vi "Bertta_v06_3.vi"() -> ()   [LabVIEW 2015]
uses:
  x64/Debug/BERTTA.dll
panel:
  in  "Tab Control":T1(tab)
  in  "Description":string
  in  "Project name":string
  in  "User (initials)":string
  out "PUMP 1":bool
  out "Mettler 5":dynamicdata(graph)
  out "Temp":dynamicdata(graph)
  out "Target":dbl
  out "Scale weight":dbl
  out "Amount now":dbl
  out "Flow rate":dbl
  out "Time to target":dbl format="%<%H:%M:%S>t"
  out "Current step":dbl
  out "weightcontrol":i32
  out "timecontrol":i32
  out "target_control":i32
  in  "Balances":bool[](array[boolean])
  out "Waveform Chart 3":dynamicdata(graph)
  out "Table":string[][](table)
  in  "Headers":string[](array[string])
  out "Boolean 12":bool
  out "Boolean 7":bool
  out "Boolean 6":bool
  out "Boolean 5":bool
  out "Boolean 4":bool
  in  "?":bool
  in  "Seq":dbl[][](array[numeric])=[[20.0, 45.0, 50.0], [46.0, 50.0, 20.0], [3.0, 3.0, 3.0]]
  out "T control":dbl
  out "Tr":dbl
  out "Tj in":dbl
  out "Tj out":dbl
  out "DT":dbl
  out "Current step":i32
  out "Elapsed":i32
  in  "Tbypass":dbl=20.0
  in  "Tfail":dbl=22.0
  in  "err":i32
  in  "PAUSE":bool
  out "Tinit":dbl
  out "Tset":dbl
  out "Time limit":dbl
  out "Waveform Chart":dynamicdata(graph)
  in  "Lauda port":dbl=9.0
  in  "Port":i32=10
  in  "Radio Buttons":enum32{"Reglo Digital", "Reglo Analog", "PAM"}(radio)
  out "Speed":dbl
  out "mA":dbl format="%#_2g"
  in  "Port":i32=15
  out "RPM":dbl format="%#_2g"
  out "Boolean 18":bool
  out "Boolean 17":bool
  out "Boolean 16":bool
  out "Boolean 15":bool
  out "Boolean 14":bool
  out "Boolean 13":bool
  out "Boolean 11":bool
  out "Boolean 10":bool
  out "Boolean 9":bool
  out "Boolean 8":bool
  in  "Seq 2":dbl[][](array[numeric])=[[3.0, 3.0, 7.0], [2.0, 2.0, 2.0], [4.0, 2.0, 100.0]]
  in  "?":bool
  out "Flow rate (g/min)":dbl
  out "Time (min)":dbl
  out "Target (g)":dbl
  out "Scale reading (g)":dbl
  out "Amount now (g)":dbl
  out "Time to target (min)":dbl format="%<%H:%M:%S>t"
  in  "Bypass (g/min)":dbl
  out "Waveform Chart 2":dynamicdata(graph)
  in  "?":bool
  out "RPM":dbl
  out "Torque":dbl
  in  "Set RPM":dbl(slide) scale=0.0..500.0
  out "Waveform Chart 4":dynamicdata(graph)
  in  "?":T2(tab)
  in  "Device port":dbl=13.0
  # "1"
  # "2"
  # "3"
  # "4"
  # "Tinit     >    Tset       min. time"
  # "Grams    /   min"
  # "Pump configuration"
  # "Scale configuration"
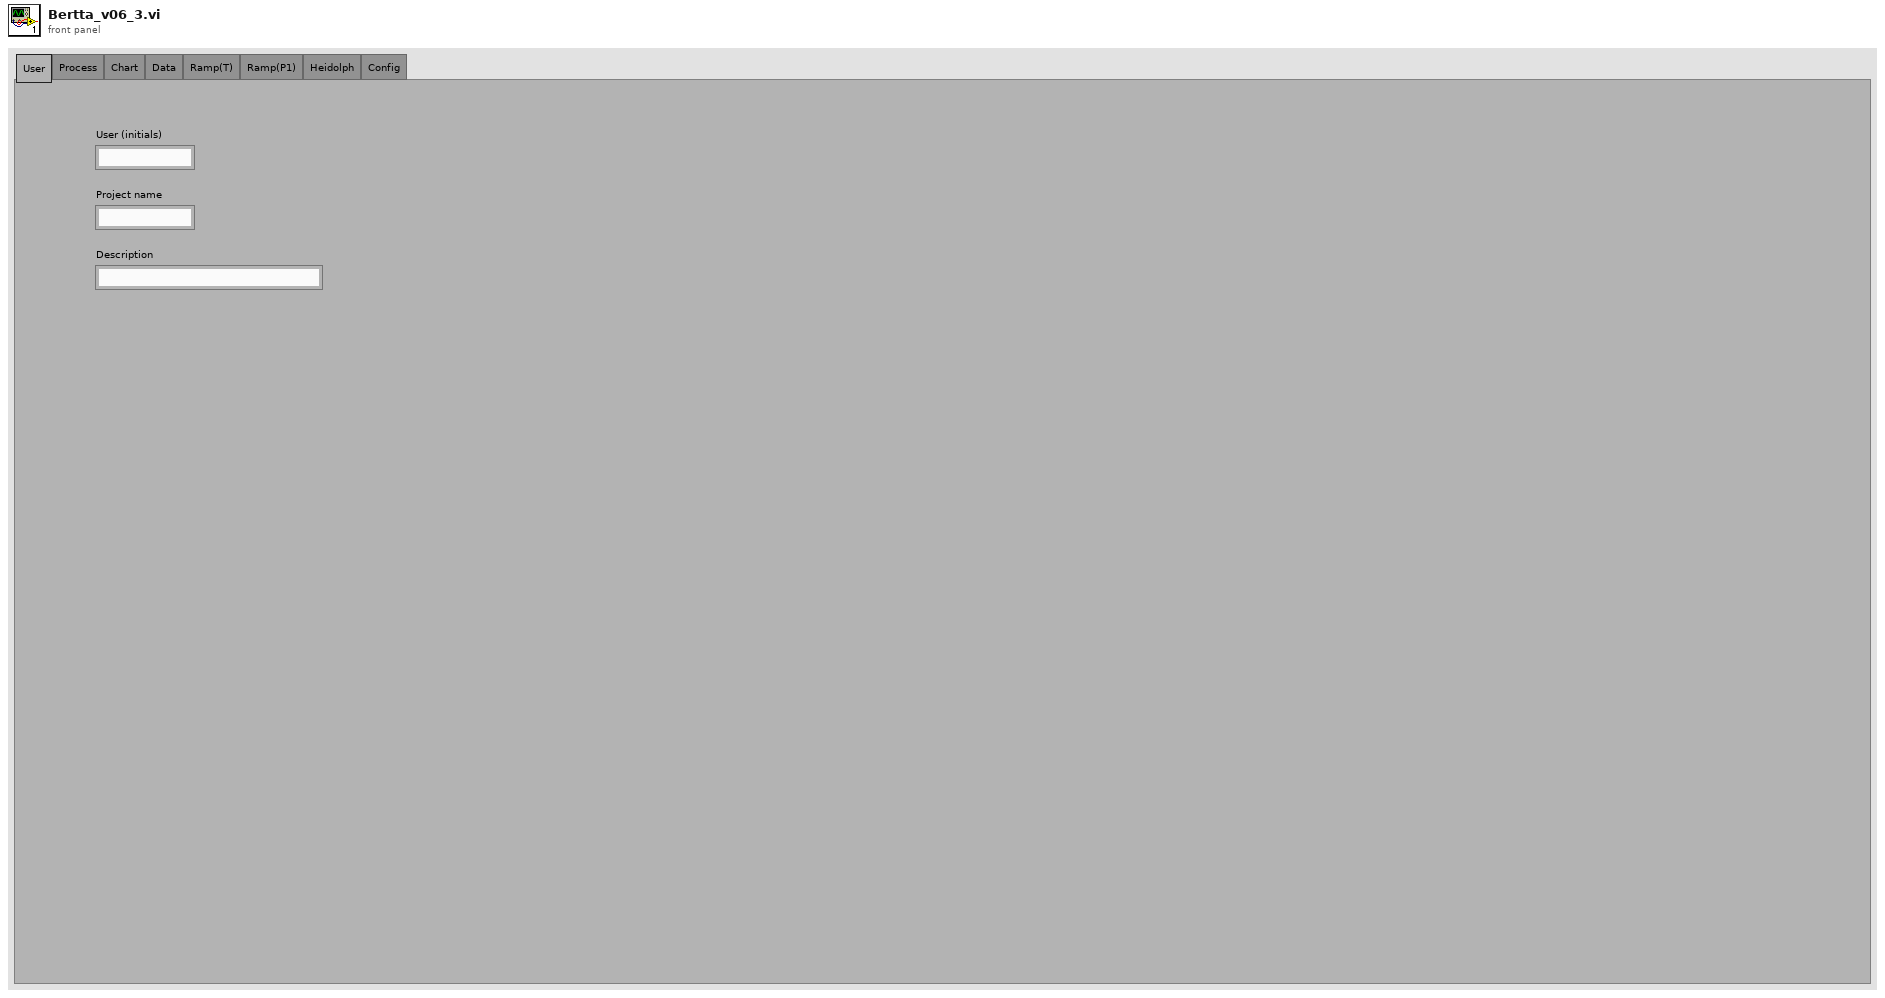
[diagram p1: front panel]
types:
  T1 = enum32{"User", "Process", "Chart", "Data", "Ramp(T)", "Ramp(P1)", "Heidolph", "Config"}
  T2 = enum32{"DB / File", "Lauda", "Heidolph", "Mettler 1", "Mettler 2", "Mettler 3", "Ismatec 1"}
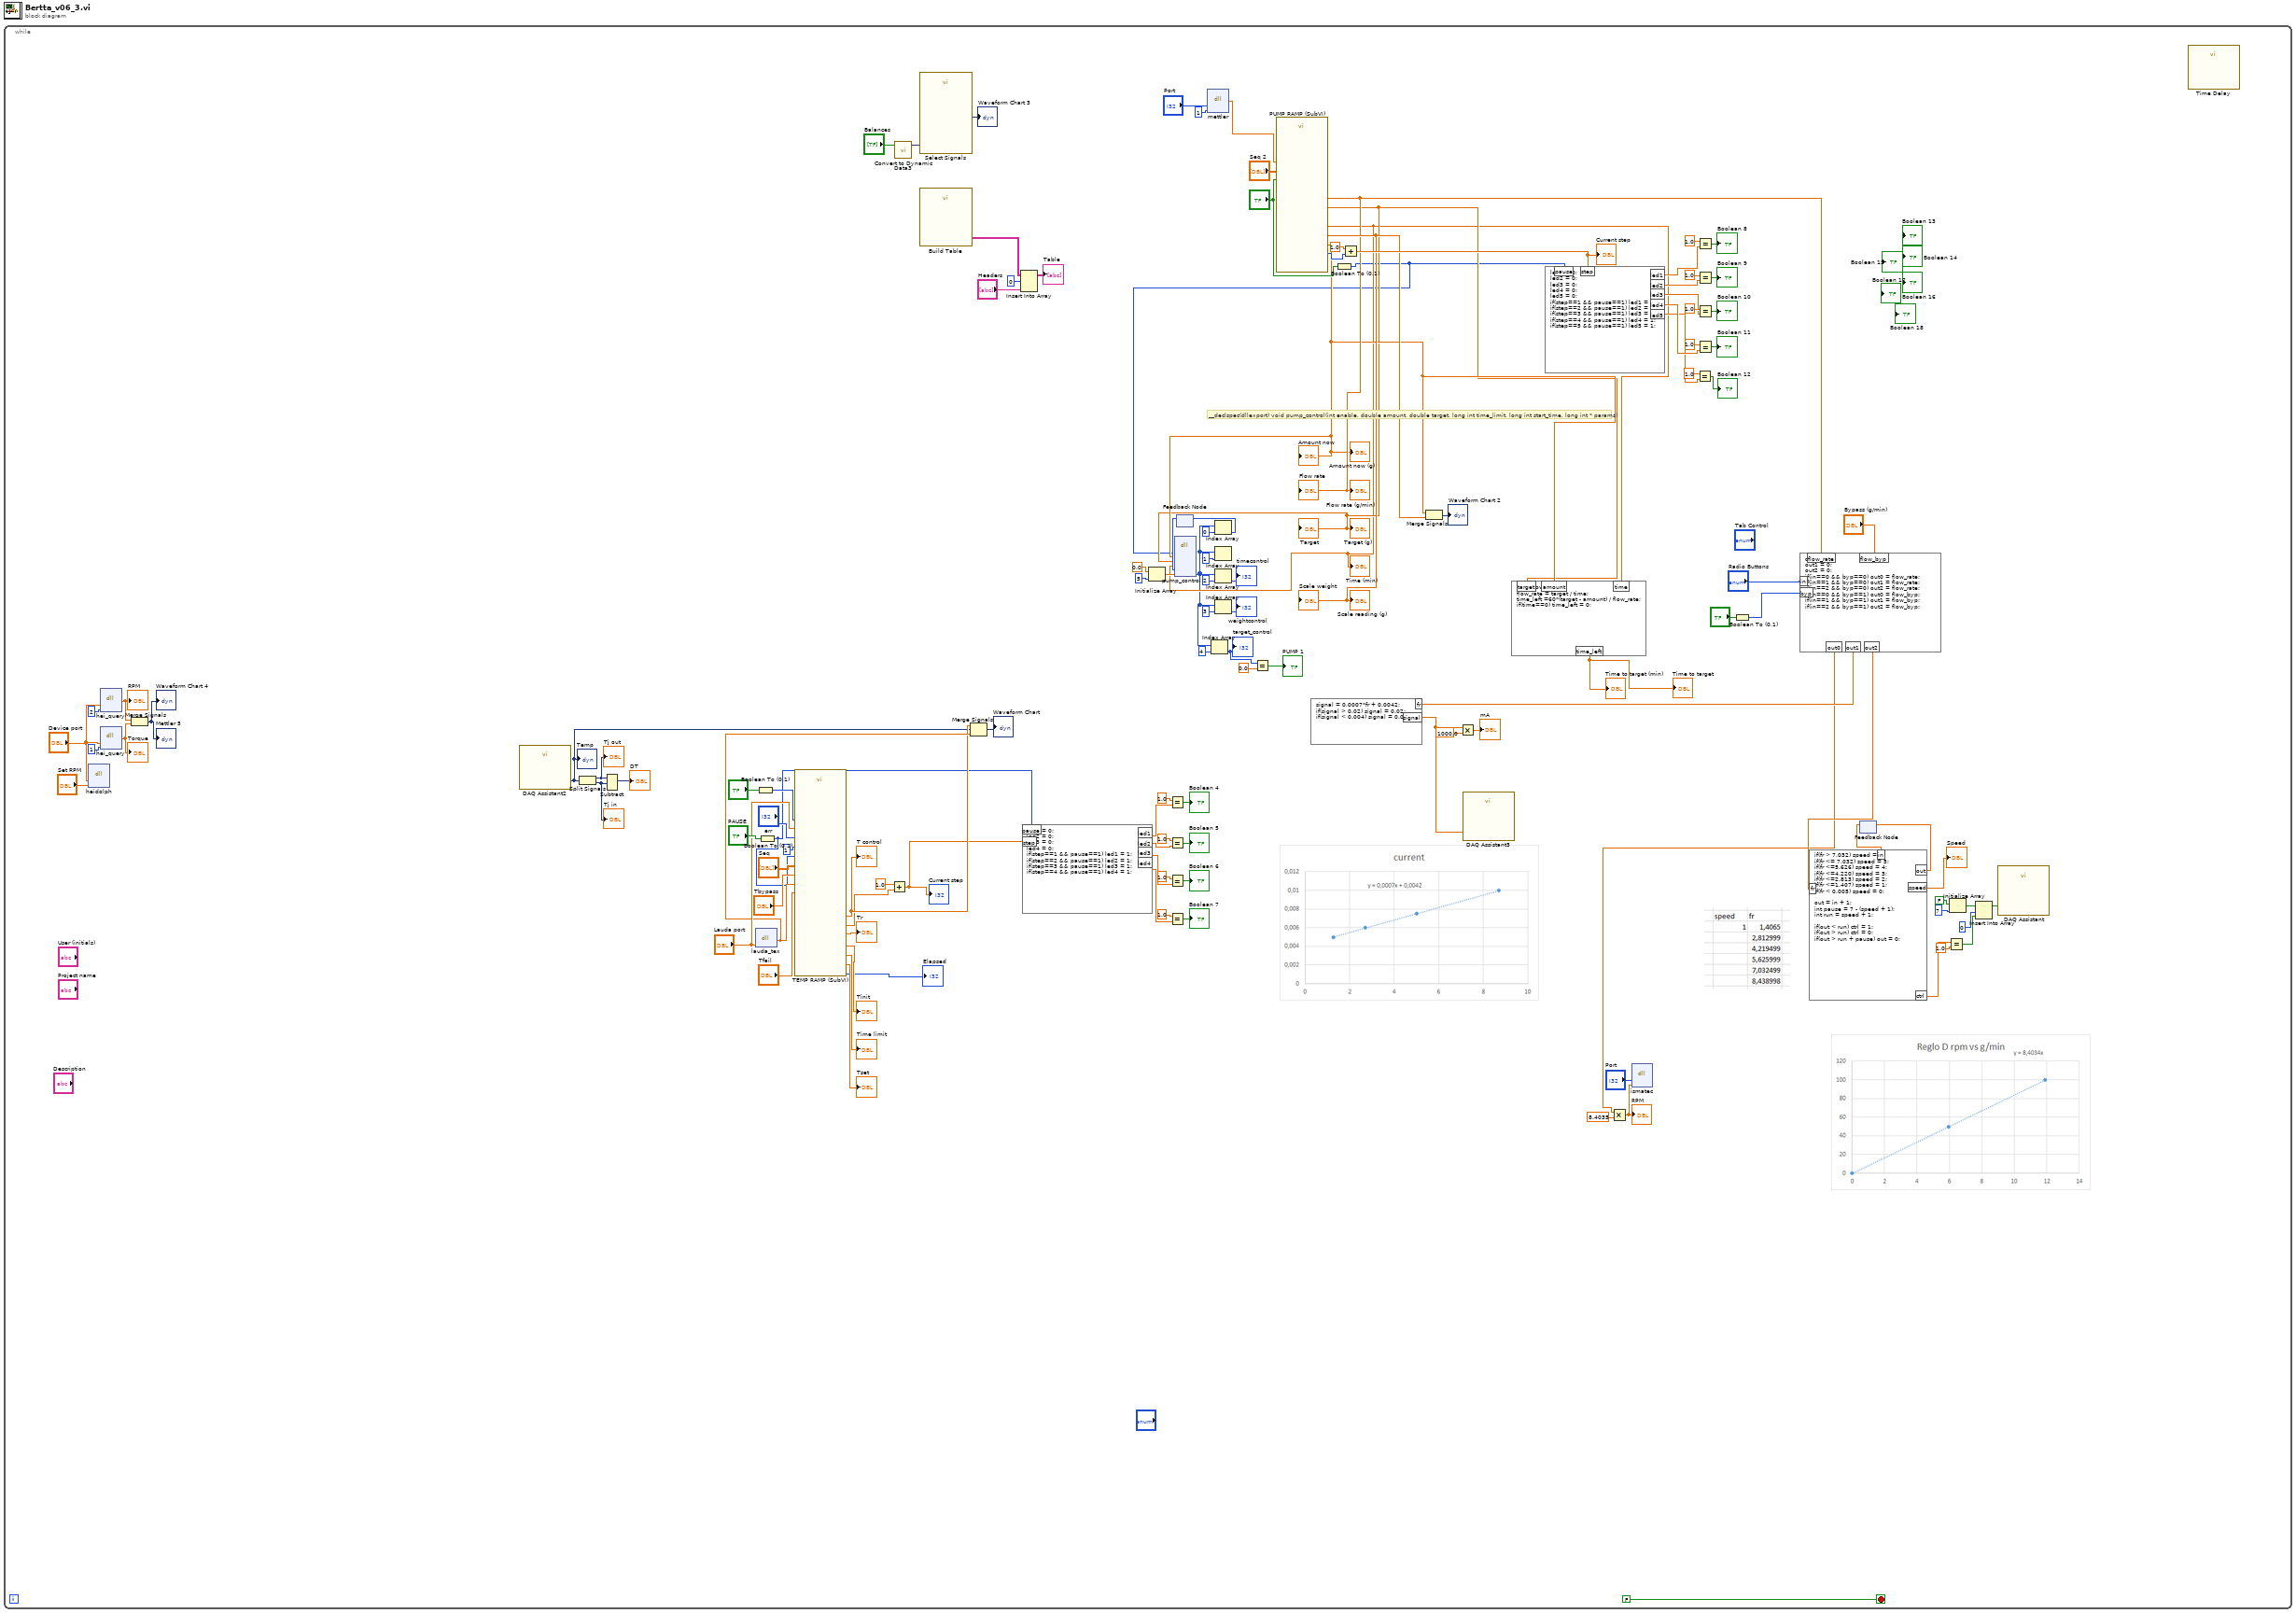
[diagram p0: block diagram]
diagram:
  n1 = while {
    stop <- FALSE stop-if-true
    # "__declspec(dllexport) void pump_control(int enable, double amount, double target, long int time_limit, long int start_time, long int * params)"
    n2 = dll-call lib="C:/Users/shresplab/OneDrive - Kemira Oyj/Documents/Visual Studio 2017/Projects/Bertta/BERTTA/x64/Debug/BERTTA.dll" fn="heidolph"("port"="Device port", "speed"="Set RPM") -> ()  [unwired: 6 in, 2 out]
    n3 = dll-call lib="C:/Users/shresplab/OneDrive - Kemira Oyj/Documents/Visual Studio 2017/Projects/Bertta/BERTTA/x64/Debug/BERTTA.dll" fn="hei_query"("port"="Device port", "q"=2) -> ("return type"=w110:dbl)  [unwired: 5 in, 2 out]
    "RPM" <- w110
    n4 = dll-call lib="C:/Users/shresplab/OneDrive - Kemira Oyj/Documents/Visual Studio 2017/Projects/Bertta/BERTTA/x64/Debug/BERTTA.dll" fn="hei_query"("port"="Device port", "q"=1) -> ("return type"=w109:dbl)  [unwired: 5 in, 2 out]
    "Torque" <- w109
    n5 = Merge Signals(w110, w109) -> (→"Waveform Chart 4" →"Mettler 5":dynamicdata)
    n6 = call "DAQ Assistant2"() -> ("data"=w26:dynamicdata)  [unwired: 17 in, 2 out]
    "Temp" <- w26
    n7 = Split Signals(w26) -> (w24:dynamicdata, w25:dynamicdata)  [unwired: 2 in]
    "Tj in" <- w25
    "Tj out" <- w24
    n8 = Subtract(1:w25, 2:w24) -> (0:→"DT":dynamicdata)  [unwired: 1 in, 1 out]
    n9 = dll-call lib="C:/Users/shresplab/OneDrive - Kemira Oyj/Documents/Visual Studio 2017/Projects/Bertta/BERTTA/x64/Debug/BERTTA.dll" fn="lauda_tex"("port"="Lauda port") -> ("return type"=w95:dbl)  [unwired: 4 in, 2 out]
    n10 = Boolean To (0,1)(Boolean="?") -> (0, 1=w101:i16)
    n11 = Boolean To (0,1)(Boolean="PAUSE") -> (0, 1=w74:i16)
    n12 = call "TEMP RAMP (SubVI).vi"("Device port"="Lauda port", "enable"=i16 1 ("Numeric"), "Tbyp"="Tbypass", "pause"=w74, "Seq"="Seq", "Tcurrent"=w95, "bypass"=w101, "err"="err", "Tfail"="Tfail") -> ("Step out"=w89:dbl, "T"=→"Tr":dbl, "Sp"=w92:dbl, "elapsed"=→"Elapsed":i32, "tr"=→"Time limit":dbl, "Tset"=→"Tset":dbl, "Tinit"=→"Tinit":dbl)  [unwired: 3 in, 1 out]
    "T control" <- w92
    n13 = Add(x=1.0, y=w89) -> (x+y=w87:dbl)
    "Current step" <- w87
    n14 = call "Convert to Dynamic Data3"("Array"="Balances") -> ("Dynamic Data Type"=w116:dynamicdata)  [unwired: 3 in]
    n15 = call "Select Signals"("Selector Input"=w116) -> ("Signal Out"=→"Waveform Chart 3":dynamicdata)  [unwired: 9 in, 1 out]
    n16 = call "Build Table"() -> ("Table"=w119:string[][])  [unwired: 5 in, 6 out]
    n17 = Merge Signals(w92, w26, w95) -> (→"Waveform Chart":dynamicdata)
    n18 = Insert Into Array(array=w119, index (row)=0, new element="Headers") -> (→"Table":string[][])  [unwired: 1 in]
    n19 = formula code="led1 = 0;\nled2 = 0;\nled3 = 0;\nled4 = 0;\nif(step==1 && pause==1) led1 = 1;\nif(step==2 && pause==1) led2 = 1;\nif(step==3 && pause==1) led3 = 1;\nif(step==4 && pause==1) led4 = 1;"("step"=w87, "pause"=w74) -> ("led1"=w85:dbl, "led2"=w81:dbl, "led3"=w79:dbl, "led4"=w77:dbl)
    n20 = Initialize Array(0.0 ("element"), 5 ("dimension size")) -> (w18:dbl[])
    n21 = Equal?(x=1.0, y=w85) -> (x = y?=→"Boolean 4":bool)
    n22 = Equal?(x=1.0, y=w81) -> (x = y?=→"Boolean 5":bool)
    n23 = Equal?(x=1.0, y=w79) -> (x = y?=→"Boolean 6":bool)
    n24 = Equal?(x=1.0, y=w77) -> (x = y?=→"Boolean 7":bool)
    n25 = feedback #1() -> (w15:i32)  [unwired: 1 in]
    n26 = dll-call lib="C:/Users/shresplab/OneDrive - Kemira Oyj/Documents/Visual Studio 2017/Projects/Bertta/BERTTA/x64/Debug/BERTTA.dll" fn="mettler"("port"="Port", "msg"=1) -> ("return type"=w27:dbl)  [unwired: 5 in, 2 out]
    n27 = call "PUMP RAMP (SubVI).vi"("in1"=w27, "Seq in"="Seq 2", 5:"?") -> ("Step"=w59:i32, "Weight (S1)"=w23:dbl, "Amount (g)"=w11:dbl, "Time (min)"=w9:dbl, "Target (g)"=w10:dbl, "Flow rate out"=w22:dbl)  [unwired: 9 in, 2 out]
    "Target (g)" <- w10
    "Time (min)" <- w9
    "Flow rate (g/min)" <- w22
    "Scale reading (g)" <- w23
    "Amount now (g)" <- w11
    "Target" <- w10
    "Scale weight" <- w23
    "Amount now" <- w11
    "Flow rate" <- w22
    n28 = Boolean To (0,1)(Boolean="?") -> (0, 1=w6:i16)
    n29 = dll-call lib="C:/Users/shresplab/OneDrive - Kemira Oyj/Documents/Visual Studio 2017/Projects/Bertta/BERTTA/x64/Debug/BERTTA.dll" fn="pump_control"("enable"=w6, "amount"=w11, "target"=w10, "time_limit"=w9, "start_time"=w15, "params"=w18) -> ("params"=w4:i32[])  [unwired: 9 in, 2 out]
    n30 = Index Array(array=w4, index=4) -> (element=w2:i32)
    "target_control" <- w2
    n31 = Index Array(array=w4, index=0) -> (element=w16:i32)
    n32 = feedback-in #1(w16) -> ()
    n33 = Index Array(array=w4, index=1) -> ()  [unwired: 1 out]
    n34 = Index Array(array=w4, index=2) -> (element=→"timecontrol":i32)
    n35 = Index Array(array=w4, index=3) -> (element=→"weightcontrol":i32)
    n36 = Equal?(x=w2, y=0.0) -> (x = y?=→"PUMP 1":bool)
    n37 = Add(x=1.0, y=w59) -> (x+y=w60:dbl)
    "Current step" <- w60
    n38 = Merge Signals(w11, w23) -> (→"Waveform Chart 2":dynamicdata)
    n39 = formula code="float flow_rate;\nflow_rate = target / time;\ntime_left =60*(target - amount) / flow_rate;\nif(time==0) time_left = 0;"("target"=w10, "amount"=w11, "time"=w9) -> ("time_left"=→"Time to target (min)" →"Time to target":dbl)
    n40 = formula code="led1 = 0;\nled2 = 0;\nled3 = 0;\nled4 = 0;\nled5 = 0;\nif(step==1 && pause==1) led1 = 1;\nif(step==2 && pause==1) led2 = 1;\nif(step==3 && pause==1) led3 = 1;\nif(step==4 && pause==1) led4 = 1;\nif(step==5 && pause==1) led5 = 1;"("step"=w60, "pause"=w6) -> ("led1"=w73:dbl, "led2"=w70:dbl, "led3"=w68:dbl, "led4"=w66:dbl, "led5"=w30:dbl)
    n41 = Equal?(x=1.0, y=w30) -> (x = y?=→"Boolean 12":bool)
    n42 = Equal?(x=1.0, y=w73) -> (x = y?=→"Boolean 8":bool)
    n43 = Equal?(x=1.0, y=w70) -> (x = y?=→"Boolean 9":bool)
    n44 = Equal?(x=1.0, y=w68) -> (x = y?=→"Boolean 10":bool)
    n45 = Equal?(x=1.0, y=w66) -> (x = y?=→"Boolean 11":bool)
    n46 = Boolean To (0,1)(Boolean="?") -> (0, 1=w37:i16)
    n47 = formula code="out0 = 0;\nout1 = 0;\nout2 = 0;\nif(in==0 && byp==0) out0 = flow_rate;\nif(in==1 && byp==0) out1 = flow_rate;\nif(in==2 && byp==0) out2 = flow_rate;\nif(in==0 && byp==1) out0 = flow_byp;\nif(in==1 && byp==1) out1 = flow_byp;\nif(in==2 && byp==1) out2 = flow_byp;"("in"="Radio Buttons", "flow_rate"=w22, "flow_byp"="Bypass (g/min)", "byp"=w37) -> ("out0"=w34:dbl, "out1"=w36:dbl, "out2"=w35:dbl)
    n48 = formula code="signal = 0.0007*fr + 0.0042;\nif(signal > 0.02) signal = 0.02;\nif(signal < 0.004) signal = 0.004;"("fr"=w36) -> ("signal"=w44:dbl)
    n49 = Multiply(x=w44, y=1000.0) -> (x*y=→"mA":dbl)
    n50 = call "DAQ Assistant3"("data"=w44) -> ()  [unwired: 17 in, 2 out]
    n51 = Multiply(x=w34, y=8.4035) -> (x*y=w41:dbl)
    "RPM" <- w41
    n52 = dll-call lib="C:/Users/shresplab/OneDrive - Kemira Oyj/Documents/Visual Studio 2017/Projects/Bertta/BERTTA/x64/Debug/BERTTA.dll" fn="ismatec"("port"="Port", "speed"=w41) -> ()  [unwired: 6 in, 2 out]
    n53 = feedback #2() -> (w49:dbl)  [unwired: 1 in]
    n54 = formula code="if(fr > 7.032) speed = 6;\nif(fr <= 7.032) speed = 5;\nif(fr <=5.626) speed = 4;\nif(fr <=4.220) speed = 3;\nif(fr <=2.813) speed = 2;\nif(fr <=1.407) speed = 1;\nif(fr < 0.005) speed = 0;\n\nout = in + 1;\nint pause = 7 - (speed + 1);\nint run = speed + 1;\n\nif(out < run) ctrl = 1;\nif(out > run) ctrl = 0;\nif(out > run + pause) out = 0;"("in"=w49, "fr"=w35) -> ("out"=w50:dbl, "ctrl"=w48:dbl, "speed"=→"Speed":dbl)
    n55 = feedback-in #2(w50) -> ()
    n56 = Equal?(x=w48, y=1.0) -> (x = y?=w46:bool)
    n57 = Initialize Array(FALSE, 7 ("dimension size")) -> (w53:bool[])
    n58 = Insert Into Array(array=w53, index=0, new element=w46) -> (w51:bool[])
    n59 = call "DAQ Assistant"("data"=w51) -> ()  [unwired: 17 in, 2 out]
    n60 = call "Time Delay"() -> ()  [unwired: 11 in, 1 out]
  }
